vi "PXI-4130 Initialization VI.vi"(8 "error in (no error)":errorcluster, 10 "Custom XML":string, 11 "Device Item Ref in":T1 format="%.0x") -> (0 "error out":errorcluster, 3 "Device Item Ref out":T1 format="%.0x")   [LabVIEW 2009, in "PXI-4130 Custom Device.lvlib"]
uses:
  PXI-4130 Custom Device.lvlib
  <vilib>/NI VeriStand/Custom Device API/Custom Device Item Ref.ctl
  <vilib>/NI VeriStand/Custom Device API/Custom Device Channel.ctl
  <vilib>/NI VeriStand/Custom Device API/Custom Device Channel Type.ctl
  <vilib>/NI VeriStand/Custom Device API/Custom Device Loop Type.ctl
  PXI-4130 Global Variable.vi
  <vilib>/NI VeriStand/Custom Device API/Custom Device API.lvlib
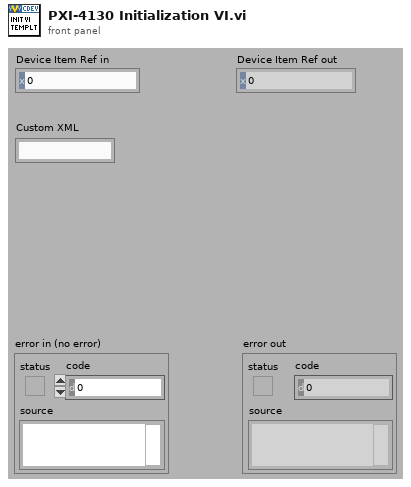
[diagram p1: front panel]
types:
  T1 = typedef "Custom Device API.lvlib/Custom Device Item Ref.ctl" = u64
  T2 = typedef "Custom Device API.lvlib/Custom Device Loop Type.ctl" = enum32{"While Loop", "Timed Loop"}
  T3 = typedef "Custom Device API.lvlib/Custom Device Channel.ctl" = cluster{"Type":T4, "Units":string, "Default Value":dbl, "Faultable":bool, "Scalable":bool}
  T4 = typedef "Custom Device API.lvlib/Custom Device Channel Type.ctl" = enum16{"Input", "Output"}
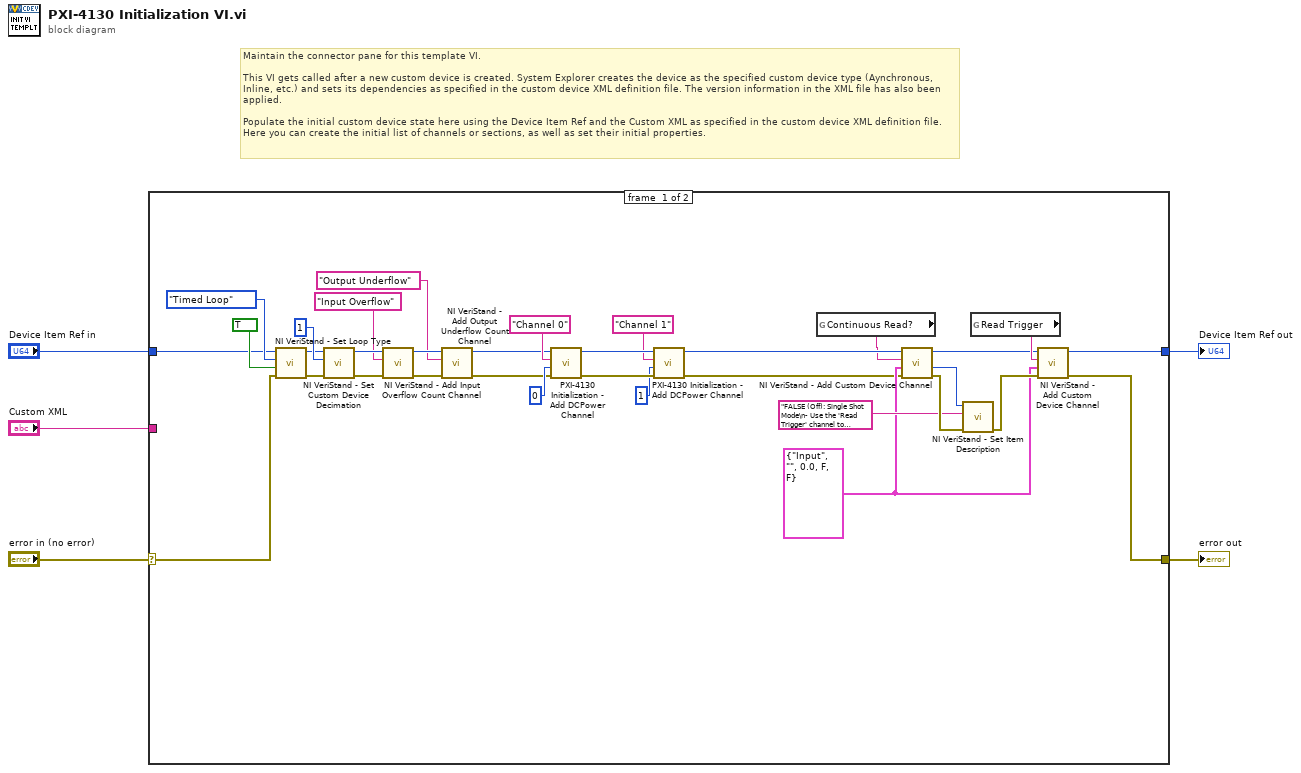
[diagram p0: block diagram]
diagram:
  # "Maintain the connector pane for this template VI.\n\nThis VI gets called after a new custom device is created. System Explorer creates the device as the specified custom device type (Aynchronous, Inline, etc.) and sets its dependencies as specified in the custom device XML definition file. The version information in the XML file has also been applied.\n\nPopulate the initial custom device state here using the Device Item Ref and the Custom XML as specified in the custom device XML definition file. Here you can create the initial list of channels or sections, as well as set their initial properties."
  n1 = case shown="No Error" "error in (no error)" {
    selector: "error in (no error)" -> [w32 w40]
    tunnel: [w15 w40] -> w5
    tunnel: [w16 w39] -> w3
    tunnel: "Device Item Ref in" -> [w33 w39]
    tunnel: "Custom XML" -> [_ _]
    frame #0 {
      w10 = T3 {"Type"=enum."Input", "Units"="", "Default Value"=0.0, "Faultable"=FALSE, "Scalable"=FALSE} ("Channel")
      n2 = call <vilib>:"NI VeriStand - Set Loop Type.vi"("error in (no error)"=w32, "Use Device Clock (Timed Loops only)"=TRUE, "Loop type"=Custom_Device_Loop_Type."Timed Loop", "Device Ref in"=w33) -> ("error out"=w36:errorcluster, "Device Ref out"=w37:T1)  [unwired: 6 in]
      n3 = call <vilib>:"NI VeriStand - Set Custom Device Decimation.vi"("error in (no error)"=w36, "Decimation"=1, "Device Ref in"=w37) -> ("error out"=w31:errorcluster, "Device Ref out"=w29:T1)  [unwired: 7 in]
      n4 = call <vilib>:"NI VeriStand - Add Input Overflow Count Channel.vi"("error in (no error)"=w31, "Channel Name"="Input Overflow", "Parent Ref in"=w29) -> ("error out"=w30:errorcluster, "Parent Ref out"=w28:T1)  [unwired: 6 in, 1 out]
      n5 = call <vilib>:"NI VeriStand - Add Output Underflow Count Channel.vi"("error in (no error)"=w30, "Channel Name"="Output Underflow", "Parent Ref in"=w28) -> ("error out"=w18:errorcluster, "Parent Ref out"=w19:T1)  [unwired: 6 in, 1 out]
      n6 = call "PXI-4130 Initialization - Add DCPower Channel.vi"("error in (no error)"=w18, "Channel #"=0, "Channel Name"="Channel 0", "Device Item Ref In"=w19) -> ("error out"=w23:errorcluster, "Device Item Ref Out"=w24:T1)  [unwired: 6 in]
      n7 = call "PXI-4130 Initialization - Add DCPower Channel.vi"("error in (no error)"=w23, "Channel #"=1, "Channel Name"="Channel 1", "Device Item Ref In"=w24) -> ("error out"=w8:errorcluster, "Device Item Ref Out"=w9:T1)  [unwired: 6 in]
      n8 = global read "PXI-4130 Global Variable.vi" "Continuous Read?"() -> (w6:string)
      n9 = call <vilib>:"NI VeriStand - Add Custom Device Channel.vi"("error in (no error)"=w8, "Channel"=w10, "Channel Name"=w6, "Parent Ref in"=w9) -> ("error out"=w13:errorcluster, "Channel Ref"=w14:T1, "Parent Ref out"=w7:T1)  [unwired: 5 in]
      n10 = call <vilib>:"NI VeriStand - Set Item Description.vi"("error in (no error)"=w13, "Description"="FALSE (Off): Single Shot Mode\n- Use the 'Read Trigger' channel to execute a single read from the SMU\nTRUE (On): Continuous Read\n- 'Read Trigger' channel is invalid" ("Units"), "Item Ref in"=w14) -> ("error out"=w12:errorcluster)  [unwired: 6 in, 2 out]
      n11 = global read "PXI-4130 Global Variable.vi" "Read Trigger"() -> (w17:string)
      n12 = call <vilib>:"NI VeriStand - Add Custom Device Channel.vi"("error in (no error)"=w12, "Channel"=w10, "Channel Name"=w17, "Parent Ref in"=w7) -> ("error out"=w15:errorcluster, "Parent Ref out"=w16:T1)  [unwired: 5 in, 1 out]
    }
    frame #1 {
    }
  }
  "error out" <- w5
  "Device Item Ref out" <- w3
